vi "Compute Watershed.vi"(8 "error in (no error)":errorcluster, 9 "Connectivity 4/8 (4)":bool=TRUE, 11 "Video Cam Processor in":refnum<class "Video Cam Processor.lvclass">) -> (0 "error out":errorcluster, 2 "Image dest. out":T1, 3 "Video Cam Processor out":refnum<class "Video Cam Processor.lvclass">)   [LabVIEW 2018, in "Video Cam Processor.lvclass"]
uses:
  Video Cam Processor.lvclass
  C:/Users/aaron.jencks/Documents/GitHub/emerson_seed_object_detection/LabVIEW/Projects/Paul's Video Viewer/Classes/Video File/Video File.lvclass
  <vilib>/vision/Image Controls.llb/IMAQ Image.ctl
  Video Cam Processor.lvclass/Video Cam Processor.ctl
  Video Frame/Video Frame.lvclass
  Video File/Video File.lvclass
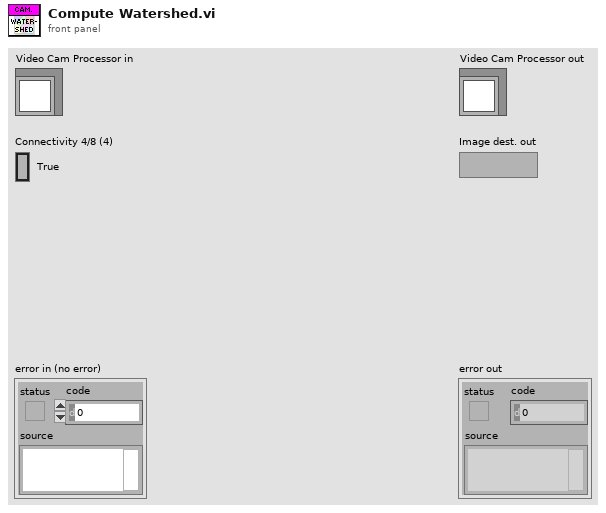
[diagram p1: front panel]
types:
  T1 = typedef "IMAQ Image.ctl" = refnum<image>
  T2 = cluster{"Area":dbl, "Number of Holes":dbl, "Bounding Rect":cluster{"Left":dbl, "Top":dbl, "Right":dbl, "Bottom":dbl}, "Center of Mass":cluster{"X":dbl, "Y":dbl}, "Orientation":dbl, "Dimensions":cluster{"Width":dbl, "Height":dbl}}[]
  T3 = cluster{"Image Dst Out":T1, "Number of Zones":i32, "Particle Reports (Pixels)":cluster{"Area":dbl, "Number of Holes":dbl, "Bounding Rect":cluster{"Left":dbl, "Top":dbl, "Right":dbl, "Bottom":dbl}, "Center of Mass":cluster{"X":dbl, "Y":dbl}, "Orientation":dbl, "Dimensions":cluster{"Width":dbl, "Height":dbl}}[]}
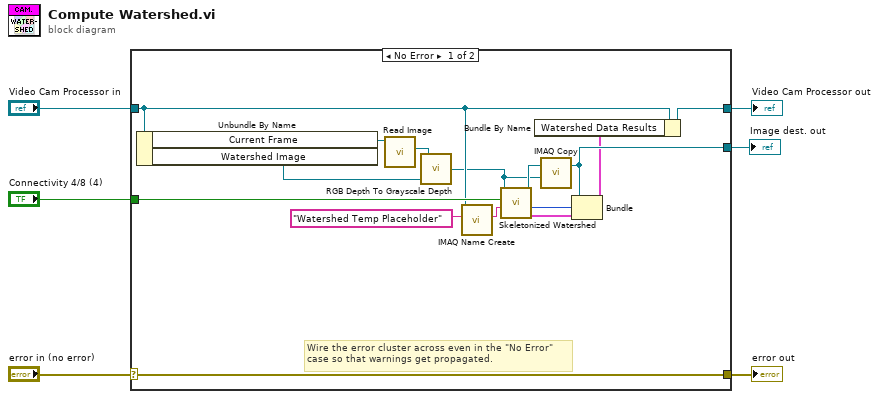
[diagram p0: block diagram]
diagram:
  n1 = case shown="No Error" "error in (no error)" {
    selector: "error in (no error)" -> [w16 w23]
    tunnel: [w16 w23] -> w5
    tunnel: [w19 w22] -> w3
    tunnel: "Video Cam Processor in" -> [w15 w22]
    tunnel: "Connectivity 4/8 (4)" -> [w17 _]
    tunnel: [w10 _] -> w1
    frame No Error {
      # "Wire the error cluster across even in the \"No Error\"\ncase so that warnings get propagated."
      n2 = Unbundle By Name(w15) -> ("Current Frame"=w21:refnum<class "Video Frame.lvclass">, "Watershed Image"=w18:T1)
      n3 = call-dynamic "Read Image.vi"("Video Frame in"=w21) -> ("Image"=w20:T1)  [unwired: 8 in, 2 out]
      n4 = call "RGB Depth To Grayscale Depth.vi"("Image Dest."=w18, "RGB Depth Image"=w20) -> ("Grayscale Depth Image"=w11:T1)  [unwired: 1 in]
      n5 = call "IMAQ Name Create.vi"("Name (\"\")"="Watershed Temp Placeholder" ("Name (\"\")"), "Video File in"=w15) -> ("Name Out"=w14:string)  [unwired: 7 in, 2 out]
      n6 = call "Skeletonized Watershed.vi"("Image Name"=w14, "Connectivity 4/8 (4)"=w17, "Grayscale Image"=w11) -> ("Particle Reports (Pixels)"=w8:T2, "Number of Zones"=w9:i32, "Image Out"=w12:T1)  [unwired: 6 in]
      n7 = call "IMAQ Copy"("Image Dst"=w11, "Image Src"=w12) -> ("Image Dst Out"=w10:T1)  [unwired: 4 in, 1 out]
      n8 = Bundle("Image Dst Out"=w10, "Number of Zones"=w9, "Particle Reports (Pixels)"=w8) -> (w7:T3)  [unwired: 1 in]
      n9 = Bundle By Name(cluster=w15, "Watershed Data Results"=w7) -> (w19:refnum<class "Video Cam Processor.lvclass">)
    }
    frame Error {
    }
  }
  "error out" <- w5
  "Video Cam Processor out" <- w3
  "Image dest. out" <- w1
